vi "rsidr_core_global.vi"() -> ()   [LabVIEW 2020, in "Rohde&Schwarz CMWXP NR FR1 Measurement.lvlib"] (continued)
command(s):\nCONFigure:NRSub:MEAS<i>:MEValuation:LIMit:PDYNamics:OFFPower"}, {"Level"=4, "Class Only"=FALSE, "Identifier"="RSCMWXPNRFR1M_ATTR_MULTI_EVAL_MEAS_LIMIT_POWER_DYNAMICS_TEST_TOLERANCES", "Descriptive Name"="Multi Eval Meas Limit Power Dynamics Test Tolerances", "Data Type"=enum."RawString", "Command"="CONF:NRS:MEAS{instance}:MEV:LIM:PDYN:TTOL:CBGT", "Access"=enum."Read/Write", "Range Table"="", "Read Callback"="", "Write Callback"="", "Range Callback"="", "Check Callback"="", "Rngtable Callback"="", "Coerce Callback"="", "Supported Models"="", "Instrument Options"="", "Check Status Callback"="", "Flags"=0, "Help"="Defines test tolerances for power dynamics limits, for channel BW > 40 MHz.\n\nSyntax:\nCONFigure:NRSub:MEAS<i>:MEValuation:LIMit:PDYNamics:TTOLerance:CBGT <TTPowerLess3G>, <TTPowerGreat3G>\n\n<TTPowerLess3G>\nFor carrier center frequencies up to 3 GHz\nValid Values:\n-3 dB to 3 dB\n\n<TTPowerGreat3G>\nFor carrier center frequencies > 3 GHz\nValid Values:\n-3 dB to 3 dB\n\nAvailable Repeated Capabilities:\ninstance: i0, i1, i2, i3, i4, i5, i6, i7, i8, i9, i10, i11, i12, i13, i14, i15, i16, i17, i18, i19, i20, i21, i22, i23, i24, i25, i26, i27, i28, i29, i30, i31, i32\r\n\nRemote-control command(s):\nCONFigure:NRSub:MEAS<i>:MEValuation:LIMit:PDYNamics:TTOLerance:CBGT"}, {"Level"=4, "Class Only"=FALSE, "Identifier"="RSCMWXPNRFR1M_ATTR_MULTI_EVAL_MEAS_LIMIT_POWER_DYNAMICS_TEST_TOLERANCES_FOR_CHANNEL_BW", "Descriptive Name"="Multi Eval Meas Limit Power Dynamics Test Tolerances For Channel BW", "Data Type"=enum."RawString", "Command"="CONF:NRS:MEAS{instance}:MEV:LIM:PDYN:TTOL:CBLT", "Access"=enum."Read/Write", "Range Table"="", "Read Callback"="", "Write Callback"="", "Range Callback"="", "Check Callback"="", "Rngtable Callback"="", "Coerce Callback"="", "Supported Models"="", "Instrument Options"="", "Check Status Callback"="", "Flags"=0, "Help"="Defines test tolerances for power dynamics limits, for channel BW up to 40 MHz.\n\nSyntax:\nCONFigure:NRSub:MEAS<i>:MEValuation:LIMit:PDYNamics:TTOLerance:CBLT <TTPowerLess3G>, <TTPowerGreat3G>\n\n<TTPowerLess3G>\nFor carrier center frequencies up to 3 GHz\nValid Values:\n-3 dB to 3 dB\n\n<TTPowerGreat3G>\nFor carrier center frequencies > 3 GHz\nValid Values:\n-3 dB to 3 dB\n\nAvailable Repeated Capabilities:\ninstance: i0, i1, i2, i3, i4, i5, i6, i7, i8, i9, i10, i11, i12, i13, i14, i15, i16, i17, i18, i19, i20, i21, i22, i23, i24, i25, i26, i27, i28, i29, i30, i31, i32\r\n\nRemote-control command(s):\nCONFigure:NRSub:MEAS<i>:MEValuation:LIMit:PDYNamics:TTOLerance:CBLT"}, {"Level"=2, "Class Only"=TRUE, "Identifier"="", "Descriptive Name"="Results", "Data Type"=enum."ViInt32", "Command"="", "Access"=enum."Read Only", "Range Table"="", "Read Callback"="", "Write Callback"="", "Range Callback"="", "Check Callback"="", "Rngtable Callback"="", "Coerce Callback"="", "Supported Models"="", "Instrument Options"="", "Check Status Callback"="", "Flags"=0, "Help"="The attributes in this class retrieve results for multi-evaluation measurements."}, {"Level"=3, "Class Only"=TRUE, "Identifier"="", "Descriptive Name"="Detected Signal Configuration", "Data Type"=enum."ViInt32", "Command"="", "Access"=enum."Read Only", "Range Table"="", "Read Callback"="", "Write Callback"="", "Range Callback"="", "Check Callback"="", "Rngtable Callback"="", "Coerce Callback"="", "Supported Models"="", "Instrument Options"="", "Check Status Callback"="", "Flags"=0, "Help"="The commands in this class return the detected allocation and modulation scheme and the view filter throughput."}, {"Level"=4, "Class Only"=FALSE, "Identifier"="RSCMWXPNRFR1M_ATTR_FETCH_MULTI_EVAL_MEAS_MODULATION_DETECTED_ALLOCATION_RESULTS", "Descriptive Name"="Fetch Multi Eval Meas Modulation Detected Allocation Results", "Data Type"=enum."RawString", "Command"="FETC:NRS:MEAS{instance}:MEV:MOD:DALL?", "Access"=enum."Read Only", "Range Table"="", "Read Callback"="", "Write Callback"="", "Range Callback"="", "Check Callback"="", "Rngtable Callback"="", "Coerce Callback"="", "Supported Models"="", "Instrument Options"="", "Check Status Callback"="", "Flags"=0, "Help"="Returns the modulation detected allocation for the measured slot.\n\nIf the same slot is measured by the individual measurements, all commands yield the same result. If different statistic counts are defined for the modulation, ACLR and spectrum emission mask measurements, different slots can be measured and different results can be returned by the individual commands.\n\nReturn values:\n<Reliability>\n decimal\n\n<NrResBlocks>\n decimal\nNumber of allocated resource blocks\n\n<OffsetResBlocks>\n decimal\nOffset of the first allocated resource block from the edge of the allocated UL transmission bandwidth\n\nAvailable Repeated Capabilities:\ninstance: i0, i1, i2, i3, i4, i5, i6, i7, i8, i9, i10, i11, i12, i13, i14, i15, i16, i17, i18, i19, i20, i21, i22, i23, i24, i25, i26, i27, i28, i29, i30, i31, i32\r\n\nRemote-control command(s):\nFETCh:NRSub:MEAS<i>:MEValuation:MODulation:DALLocation?"}, {"Level"=4, "Class Only"=FALSE, "Identifier"="RSCMWXPNRFR1M_ATTR_FETCH_MULTI_EVAL_MEAS_MODULATION_DETECTED_MODULATION_RESULTS", "Descriptive Name"="Fetch Multi Eval Meas Modulation Detected Modulation Results", "Data Type"=enum."RawString", "Command"="FETC:NRS:MEAS{instance}:MEV:MOD:DMOD?", "Access"=enum."Read Only", "Range Table"="", "Read Callback"="", "Write Callback"="", "Range Callback"="", "Check Callback"="", "Rngtable Callback"="", "Coerce Callback"="", "Supported Models"="", "Instrument Options"="", "Check Status Callback"="", "Flags"=0, "Help"="Returns the detected modulation scheme in the measured slot.\n\nReturn values:\n<Reliability>\n decimal\n\n<Modulation>\n BPSK | BPWS | QPSK | Q16 | Q64 | Q256\nBPSK, BPWS: Pi/2-BPSK, Pi/2-BPSK with shaping\nQPSK, Q16, Q64, Q256: QPSK, 16-QAM, 64-QAM, 256-QAM\n\nAvailable Repeated Capabilities:\ninstance: i0, i1, i2, i3, i4, i5, i6, i7, i8, i9, i10, i11, i12, i13, i14, i15, i16, i17, i18, i19, i20, i21, i22, i23, i24, i25, i26, i27, i28, i29, i30, i31, i32\r\n\nRemote-control command(s):\nFETCh:NRSub:MEAS<i>:MEValuation:MODulation:DMODulation?"}, {"Level"=4, "Class Only"=FALSE, "Identifier"="RSCMWXPNRFR1M_ATTR_FETCH_MULTI_EVAL_MEAS_ACLR_DETECTED_ALLOCATION_RESULTS", "Descriptive Name"="Fetch Multi Eval Meas ACLR Detected Allocation Results", "Data Type"=enum."RawString", "Command"="FETC:NRS:MEAS{instance}:MEV:ACLR:DALL?", "Access"=enum."Read Only", "Range Table"="", "Read Callback"="", "Write Callback"="", "Range Callback"="", "Check Callback"="", "Rngtable Callback"="", "Coerce Callback"="", "Supported Models"="", "Instrument Options"="", "Check Status Callback"="", "Flags"=0, "Help"="Returns the ACLR detected allocation for the measured slot.\n\nIf the same slot is measured by the individual measurements, all commands yield the same result. If different statistic counts are defined for the modulation, ACLR and spectrum emission mask measurements, different slots can be measured and different results can be returned by the individual commands.\n\nReturn values:\n<Reliability>\n decimal\n\n<NrResBlocks>\n decimal\nNumber of allocated resource blocks\n\n<OffsetResBlocks>\n decimal\nOffset of the first allocated resource block from the edge of the allocated UL transmission bandwidth\n\nAvailable Repeated Capabilities:\ninstance: i0, i1, i2, i3, i4, i5, i6, i7, i8, i9, i10, i11, i12, i13, i14, i15, i16, i17, i18, i19, i20, i21, i22, i23, i24, i25, i26, i27, i28, i29, i30, i31, i32\r\n\nRemote-control command(s):\nFETCh:NRSub:MEAS<i>:MEValuation:ACLR:DALLocation?"}, {"Level"=4, "Class Only"=FALSE, "Identifier"="RSCMWXPNRFR1M_ATTR_FETCH_MULTI_EVAL_MEAS_SEM_DETECTED_ALLOCATION_RESULTS", "Descriptive Name"="Fetch Multi Eval Meas SEM Detected Allocation Results", "Data Type"=enum."RawString", "Command"="FETC:NRS:MEAS{instance}:MEV:SEM:DALL?", "Access"=enum."Read Only", "Range Table"="", "Read Callback"="", "Write Callback"="", "Range Callback"="", "Check Callback"="", "Rngtable Callback"="", "Coerce Callback"="", "Supported Models"="", "Instrument Options"="", "Check Status Callback"="", "Flags"=0, "Help"="Returns the spectrum emission mask detected allocation for the measured slot.\n\nIf the same slot is measured by the individual measurements, all commands yield the same result. If different statistic counts are defined for the modulation, ACLR and spectrum emission mask measurements, different slots can be measured and different results can be returned by the individual commands.\n\nReturn values:\n<Reliability>\n decimal\n\n<NrResBlocks>\n decimal\nNumber of allocated resource blocks\n\n<OffsetResBlocks>\n decimal\nOffset of the first allocated resource block from the edge of the allocated UL transmission bandwidth\n\nAvailable Repeated Capabilities:\ninstance: i0, i1, i2, i3, i4, i5, i6, i7, i8, i9, i10, i11, i12, i13, i14, i15, i16, i17, i18, i19, i20, i21, i22, i23, i24, i25, i26, i27, i28, i29, i30, i31, i32\r\n\nRemote-control command(s):\nFETCh:NRSub:MEAS<i>:MEValuation:SEMask:DALLocation?"}, {"Level"=4, "Class Only"=FALSE, "Identifier"="RSCMWXPNRFR1M_ATTR_FETCH_MULTI_EVAL_MEAS_VIEW_FILTER_THROUGHPUT", "Descriptive Name"="Fetch Multi Eval Meas View Filter Throughput", "Data Type"=enum."RawString", "Command"="FETC:NRS:MEAS{instance}:MEV:VFTH?", "Access"=enum."Read Only", "Range Table"="", "Read Callback"="", "Write Callback"="", "Range Callback"="", "Check Callback"="", "Rngtable Callback"="", "Coerce Callback"="", "Supported Models"="", "Instrument Options"="", "Check Status Callback"="", "Flags"=0, "Help"="Queries the percentage of measurement intervals in which the detected signal configuration matched the 'View Filter' settings. Only slots which contribute to the 'View Filter Throughput' are displayed, counted, and used for the statistical results. Other slots are rejected.\n\nThe 'View Filter Throughput' is evaluated in a moving window of 1000 frames. If a non-matching signal configuration is changed according to the 'View Filter' settings, the throughput increases linearly from 0% to 100%.\n\n<Reliability>\n decimal\n'Reliability Indicator'\n\n<VFThroughput>\n float\nDefault unit:  %\n\nAvailable Repeated Capabilities:\ninstance: i0, i1, i2, i3, i4, i5, i6, i7, i8, i9, i10, i11, i12, i13, i14, i15, i16, i17, i18, i19, i20, i21, i22, i23, i24, i25, i26, i27, i28, i29, i30, i31, i32\r\n\nRemote-control command(s):\nFETCh:NRSub:MEAS<i>:MEValuation:VFTHroughput?"}, {"Level"=3, "Class Only"=TRUE, "Identifier"="", "Descriptive Name"="EVM Trace Results", "Data Type"=enum."ViInt32", "Command"="", "Access"=enum."Read Only", "Range Table"="", "Read Callback"="", "Write Callback"="", "Range Callback"="", "Check Callback"="", "Rngtable Callback"="", "Coerce Callback"="", "Supported Models"="", "Instrument Options"="", "Check Status Callback"="", "Flags"=0, "Help"="The commands in this class return the contents of the EVM result diagrams."}, {"Level"=4, "Class Only"=FALSE, "Identifier"="RSCMWXPNRFR1M_ATTR_READ_MULTI_EVAL_MEAS_EVM_CURRENT_RESULTS", "Descriptive Name"="Read Multi Eval Meas EVM Current Results", "Data Type"=enum."RawString", "Command"="READ:NRS:MEAS{instance}:MEV:EVM:CURR?", "Access"=enum."Read Only", "Range Table"="", "Read Callback"="", "Write Callback"="", "Range Callback"="", "Check Callback"="", "Rngtable Callback"="", "Coerce Callback"="", "Supported Models"="", "Instrument Options"="", "Check Status Callback"="", "Flags"=0, "Help"="Returns the values of the EVM RMS bar graphs for the OFDM symbols in the measured slot. The results of the current bar graph are retrieved.\n\nThere is one pair of EVM values per OFDM symbol, returned in the following order:\n<Reliability>, {<Low>, <High>}symbol 0, {<Low>, <High>}symbol 1, ...\n\nReturn values:\n<Reliability>\n decimal\n\n<Low>\n float\nEVM value for low EVM window position.\nDefault unit:  %\n\n<High>\n float\nEVM value for high EVM window position.\nDefault unit:  %\n\nAvailable Repeated Capabilities:\ninstance: i0, i1, i2, i3, i4, i5, i6, i7, i8, i9, i10, i11, i12, i13, i14, i15, i16, i17, i18, i19, i20, i21, i22, i23, i24, i25, i26, i27, i28, i29, i30, i31, i32\r\n\nRemote-control command(s):\nREAD:NRSub:MEAS<i>:MEValuation:EVMagnitude:CURRent?"}, {"Level"=4, "Class Only"=FALSE, "Identifier"="RSCMWXPNRFR1M_ATTR_READ_MULTI_EVAL_MEAS_EVM_AVERAGE_RESULTS", "Descriptive Name"="Read Multi Eval Meas EVM Average Results", "Data Type"=enum."RawString", "Command"="READ:NRS:MEAS{instance}:MEV:EVM:AVER?", "Access"=enum."Read Only", "Range Table"="", "Read Callback"="", "Write Callback"="", "Range Callback"="", "Check Callback"="", "Rngtable Callback"="", "Coerce Callback"="", "Supported Models"="", "Instrument Options"="", "Check Status Callback"="", "Flags"=0, "Help"="Returns the values of the EVM RMS bar graphs for the OFDM symbols in the measured slot. The results of the average  bar graph are retrieved.\n\nThere is one pair of EVM values per OFDM symbol, returned in the following order:\n<Reliability>, {<Low>, <High>}symbol 0, {<Low>, <High>}symbol 1, ...\n\nReturn values:\n<Reliability>\n decimal\n\n<Low>\n float\nEVM value for low EVM window position.\nDefault unit:  %\n\n<High>\n float\nEVM value for high EVM window position.\nDefault unit:  %\n\nAvailable Repeated Capabilities:\ninstance: i0, i1, i2, i3, i4, i5, i6, i7, i8, i9, i10, i11, i12, i13, i14, i15, i16, i17, i18, i19, i20, i21, i22, i23, i24, i25, i26, i27, i28, i29, i30, i31, i32\r\n\nRemote-control command(s):\nREAD:NRSub:MEAS<i>:MEValuation:EVMagnitude:AVERage?"}, {"Level"=4, "Class Only"=FALSE, "Identifier"="RSCMWXPNRFR1M_ATTR_READ_MULTI_EVAL_MEAS_EVM_MAXIMUM_RESULTS", "Descriptive Name"="Read Multi Eval Meas EVM Maximum Results", "Data Type"=enum."RawString", "Command"="READ:NRS:MEAS{instance}:MEV:EVM:MAX?", "Access"=enum."Read Only", "Range Table"="", "Read Callback"="", "Write Callback"="", "Range Callback"="", "Check Callback"="", "Rngtable Callback"="", "Coerce Callback"="", "Supported Models"="", "Instrument Options"="", "Check Status Callback"="", "Flags"=0, "Help"="Returns the values of the EVM RMS bar graphs for the OFDM symbols in the measured slot. The results of the maximum bar graph are retrieved.\n\nThere is one pair of EVM values per OFDM symbol, returned in the following order:\n<Reliability>, {<Low>, <High>}symbol 0, {<Low>, <High>}symbol 1, ...\n\nReturn values:\n<Reliability>\n decimal\n\n<Low>\n float\nEVM value for low EVM window position.\nDefault unit:  %\n\n<High>\n float\nEVM value for high EVM window position.\nDefault unit:  %\n\nAvailable Repeated Capabilities:\ninstance: i0, i1, i2, i3, i4, i5, i6, i7, i8, i9, i10, i11, i12, i13, i14, i15, i16, i17, i18, i19, i20, i21, i22, i23, i24, i25, i26, i27, i28, i29, i30, i31, i32\r\n\nRemote-control command(s):\nREAD:NRSub:MEAS<i>:MEValuation:EVMagnitude:MAXimum?"}, {"Level"=4, "Class Only"=FALSE, "Identifier"="RSCMWXPNRFR1M_ATTR_FETCH_MULTI_EVAL_MEAS_EVM_CURRENT_RESULTS", "Descriptive Name"="Fetch Multi Eval Meas EVM Current Results", "Data Type"=enum."RawString", "Command"="FETC:NRS:MEAS{instance}:MEV:EVM:CURR?", "Access"=enum."Read Only", "Range Table"="", "Read Callback"="", "Write Callback"="", "Range Callback"="", "Check Callback"="", "Rngtable Callback"="", "Coerce Callback"="", "Supported Models"="", "Instrument Options"="", "Check Status Callback"="", "Flags"=0, "Help"="Returns the values of the EVM RMS bar graphs for the OFDM symbols in the measured slot. The results of the current bar graph are retrieved.\n\nThere is one pair of EVM values per OFDM symbol, returned in the following order:\n<Reliability>, {<Low>, <High>}symbol 0, {<Low>, <High>}symbol 1, ...\n\nReturn values:\n<Reliability>\n decimal\n\n<Low>\n float\nEVM value for low EVM window position.\nDefault unit:  %\n\n<High>\n float\nEVM value for high EVM window position.\nDefault unit:  %\n\nAvailable Repeated Capabilities:\ninstance: i0, i1, i2, i3, i4, i5, i6, i7, i8, i9, i10, i11, i12, i13, i14, i15, i16, i17, i18, i19, i20, i21, i22, i23, i24, i25, i26, i27, i28, i29, i30, i31, i32\r\n\nRemote-control command(s):\nFETCh:NRSub:MEAS<i>:MEValuation:EVMagnitude:CURRent?"}, {"Level"=4, "Class Only"=FALSE, "Identifier"="RSCMWXPNRFR1M_ATTR_FETCH_MULTI_EVAL_MEAS_EVM_AVERAGE_RESULTS", "Descriptive Name"="Fetch Multi Eval Meas EVM Average Results", "Data Type"=enum."RawString", "Command"="FETC:NRS:MEAS{instance}:MEV:EVM:AVER?", "Access"=enum."Read Only", "Range Table"="", "Read Callback"="", "Write Callback"="", "Range Callback"="", "Check Callback"="", "Rngtable Callback"="", "Coerce Callback"="", "Supported Models"="", "Instrument Options"="", "Check Status Callback"="", "Flags"=0, "Help"="Returns the values of the EVM RMS bar graphs for the OFDM symbols in the measured slot. The results of the average  bar graph are retrieved.\n\nThere is one pair of EVM values per OFDM symbol, returned in the following order:\n<Reliability>, {<Low>, <High>}symbol 0, {<Low>, <High>}symbol 1, ...\n\nReturn values:\n<Reliability>\n decimal\n\n<Low>\n float\nEVM value for low EVM window position.\nDefault unit:  %\n\n<High>\n float\nEVM value for high EVM window position.\nDefault unit:  %\n\nAvailable Repeated Capabilities:\ninstance: i0, i1, i2, i3, i4, i5, i6, i7, i8, i9, i10, i11, i12, i13, i14, i15, i16, i17, i18, i19, i20, i21, i22, i23, i24, i25, i26, i27, i28, i29, i30, i31, i32\r\n\nRemote-control command(s):\nFETCh:NRSub:MEAS<i>:MEValuation:EVMagnitude:AVERage?"}, {"Level"=4, "Class Only"=FALSE, "Identifier"="RSCMWXPNRFR1M_ATTR_FETCH_MULTI_EVAL_MEAS_EVM_MAXIMUM_RESULTS", "Descriptive Name"="Fetch Multi Eval Meas EVM Maximum Results", "Data Type"=enum."RawString", "Command"="FETC:NRS:MEAS{instance}:MEV:EVM:MAX?", "Access"=enum."Read Only", "Range Table"="", "Read Callback"="", "Write Callback"="", "Range Callback"="", "Check Callback"="", "Rngtable Callback"="", "Coerce Callback"="", "Supported Models"="", "Instrument Options"="", "Check Status Callback"="", "Flags"=0, "Help"="Returns the values of the EVM RMS bar graphs for the OFDM symbols in the measured slot. The results of the maximum bar graph are retrieved.\n\nThere is one pair of EVM values per OFDM symbol, returned in the following order:\n<Reliability>, {<Low>, <High>}symbol 0, {<Low>, <High>}symbol 1, ...\n\nReturn values:\n<Reliability>\n decimal\n\n<Low>\n float\nEVM value for low EVM window position.\nDefault unit:  %\n\n<High>\n float\nEVM value for high EVM window position.\nDefault unit:  %\n\nAvailable Repeated Capabilities:\ninstance: i0, i1, i2, i3, i4, i5, i6, i7, i8, i9, i10, i11, i12, i13, i14, i15, i16, i17, i18, i19, i20, i21, i22, i23, i24, i25, i26, i27, i28, i29, i30, i31, i32\r\n\nRemote-control command(s):\nFETCh:NRSub:MEAS<i>:MEValuation:EVMagnitude:MAXimum?"}, {"Level"=4, "Class Only"=FALSE, "Identifier"="RSCMWXPNRFR1M_ATTR_READ_MULTI_EVAL_MEAS_EVM_PEAK_CURRENT_RESULTS", "Descriptive Name"="Read Multi Eval Meas EVM Peak Current Results", "Data Type"=enum."RawString", "Command"="READ:NRS:MEAS{instance}:MEV:EVM:PEAK:CURR?", "Access"=enum."Read Only", "Range Table"="", "Read Callback"="", "Write Callback"="", "Range Callback"="", "Check Callback"="", "Rngtable Callback"="", "Coerce Callback"="", "Supported Models"="", "Instrument Options"="", "Check Status Callback"="", "Flags"=0, "Help"="Returns the values of the EVM peak bar graphs for the OFDM symbols in the measured slot. The results of the current bar graph are retrieved.\n\nThere is one pair of EVM values per OFDM symbol, returned in the following order:\n<Reliability>, {<Low>, <High>}symbol 0, {<Low>, <High>}symbol 1, ...\n\nReturn values:\n<Reliability>\n decimal\n\n<Low>\n float\nEVM value for low EVM window position.\nDefault unit:  %\n\n<High>\n float\nEVM value for high EVM window position.\nDefault unit:  %\n\nAvailable Repeated Capabilities:\ninstance: i0, i1, i2, i3, i4, i5, i6, i7, i8, i9, i10, i11, i12, i13, i14, i15, i16, i17, i18, i19, i20, i21, i22, i23, i24, i25, i26, i27, i28, i29, i30, i31, i32\r\n\nRemote-control command(s):\nREAD:NRSub:MEAS<i>:MEValuation:EVMagnitude:PEAK:CURRent?"}, {"Level"=4, "Class Only"=FALSE, "Identifier"="RSCMWXPNRFR1M_ATTR_READ_MULTI_EVAL_MEAS_EVM_PEAK_AVERAGE_RESULTS", "Descriptive Name"="Read Multi Eval Meas EVM Peak Average Results", "Data Type"=enum."RawString", "Command"="READ:NRS:MEAS{instance}:MEV:EVM:PEAK:AVER?", "Access"=enum."Read Only", "Range Table"="", "Read Callback"="", "Write Callback"="", "Range Callback"="", "Check Callback"="", "Rngtable Callback"="", "Coerce Callback"="", "Supported Models"="", "Instrument Options"="", "Check Status Callback"="", "Flags"=0, "Help"="Returns the values of the EVM peak bar graphs for the OFDM symbols in the measured slot. The results of the average bar graph are retrieved.\n\nThere is one pair of EVM values per OFDM symbol, returned in the following order:\n<Reliability>, {<Low>, <High>}symbol 0, {<Low>, <High>}symbol 1, ...\n\nReturn values:\n<Reliability>\n decimal\n\n<Low>\n float\nEVM value for low EVM window position.\nDefault unit:  %\n\n<High>\n float\nEVM value for high EVM window position.\nDefault unit:  %\n\nAvailable Repeated Capabilities:\ninstance: i0, i1, i2, i3, i4, i5, i6, i7, i8, i9, i10, i11, i12, i13, i14, i15, i16, i17, i18, i19, i20, i21, i22, i23, i24, i25, i26, i27, i28, i29, i30, i31, i32\r\n\nRemote-control command(s):\nREAD:NRSub:MEAS<i>:MEValuation:EVMagnitude:PEAK:AVERage?"}, {"Level"=4, "Class Only"=FALSE, "Identifier"="RSCMWXPNRFR1M_ATTR_READ_MULTI_EVAL_MEAS_EVM_PEAK_MAXIMUM_RESULTS", "Descriptive Name"="Read Multi Eval Meas EVM Peak Maximum Results", "Data Type"=enum."RawString", "Command"="READ:NRS:MEAS{instance}:MEV:EVM:PEAK:MAX?", "Access"=enum."Read Only", "Range Table"="", "Read Callback"="", "Write Callback"="", "Range Callback"="", "Check Callback"="", "Rngtable Callback"="", "Coerce Callback"="", "Supported Models"="", "Instrument Options"="", "Check Status Callback"="", "Flags"=0, "Help"="Returns the values of the EVM peak bar graphs for the OFDM symbols in the measured slot. The results of the maximum bar graph are retrieved.\n\nThere is one pair of EVM values per OFDM symbol, returned in the following order:\n<Reliability>, {<Low>, <High>}symbol 0, {<Low>, <High>}symbol 1, ...\n\nReturn values:\n<Reliability>\n decimal\n\n<Low>\n float\nEVM value for low EVM window position.\nDefault unit:  %\n\n<High>\n float\nEVM value for high EVM window position.\nDefault unit:  %\n\nAvailable Repeated Capabilities:\ninstance: i0, i1, i2, i3, i4, i5, i6, i7, i8, i9, i10, i11, i12, i13, i14, i15, i16, i17, i18, i19, i20, i21, i22, i23, i24, i25, i26, i27, i28, i29, i30, i31, i32\r\n\nRemote-control command(s):\nREAD:NRSub:MEAS<i>:MEValuation:EVMagnitude:PEAK:MAXimum?"}, {"Level"=4, "Class Only"=FALSE, "Identifier"="RSCMWXPNRFR1M_ATTR_FETCH_MULTI_EVAL_MEAS_EVM_PEAK_CURRENT_RESULTS", "Descriptive Name"="Fetch Multi Eval Meas EVM Peak Current Results", "Data Type"=enum."RawString", "Command"="FETC:NRS:MEAS{instance}:MEV:EVM:PEAK:CURR?", "Access"=enum."Read Only", "Range Table"="", "Read Callback"="", "Write Callback"="", "Range Callback"="", "Check Callback"="", "Rngtable Callback"="", "Coerce Callback"="", "Supported Models"="", "Instrument Options"="", "Check Status Callback"="", "Flags"=0, "Help"="Returns the values of the EVM peak bar graphs for the OFDM symbols in the measured slot. The results of the current bar graph are retrieved.\n\nThere is one pair of EVM values per OFDM symbol, returned in the following order:\n<Reliability>, {<Low>, <High>}symbol 0, {<Low>, <High>}symbol 1, ...\n\nReturn values:\n<Reliability>\n decimal\n\n<Low>\n float\nEVM value for low EVM window position.\nDefault unit:  %\n\n<High>\n float\nEVM value for high EVM window position.\nDefault unit:  %\n\nAvailable Repeated Capabilities:\ninstance: i0, i1, i2, i3, i4, i5, i6, i7, i8, i9, i10, i11, i12, i13, i14, i15, i16, i17, i18, i19, i20, i21, i22, i23, i24, i25, i26, i27, i28, i29, i30, i31, i32\r\n\nRemote-control command(s):\nFETCh:NRSub:MEAS<i>:MEValuation:EVMagnitude:PEAK:CURRent?"}, {"Level"=4, "Class Only"=FALSE, "Identifier"="RSCMWXPNRFR1M_ATTR_FETCH_MULTI_EVAL_MEAS_EVM_PEAK_AVERAGE_RESULTS", "Descriptive Name"="Fetch Multi Eval Meas EVM Peak Average Results", "Data Type"=enum."RawString", "Command"="FETC:NRS:MEAS{instance}:MEV:EVM:PEAK:AVER?", "Access"=enum."Read Only", "Range Table"="", "Read Callback"="", "Write Callback"="", "Range Callback"="", "Check Callback"="", "Rngtable Callback"="", "Coerce Callback"="", "Supported Models"="", "Instrument Options"="", "Check Status Callback"="", "Flags"=0, "Help"="Returns the values of the EVM peak bar graphs for the OFDM symbols in the measured slot. The results of the average bar graph are retrieved.\n\nThere is one pair of EVM values per OFDM symbol, returned in the following order:\n<Reliability>, {<Low>, <High>}symbol 0, {<Low>, <High>}symbol 1, ...\n\nReturn values:\n<Reliability>\n decimal\n\n<Low>\n float\nEVM value for low EVM window position.\nDefault unit:  %\n\n<High>\n float\nEVM value for high EVM window position.\nDefault unit:  %\n\nAvailable Repeated Capabilities:\ninstance: i0, i1, i2, i3, i4, i5, i6, i7, i8, i9, i10, i11, i12, i13, i14, i15, i16, i17, i18, i19, i20, i21, i22, i23, i24, i25, i26, i27, i28, i29, i30, i31, i32\r\n\nRemote-control command(s):\nFETCh:NRSub:MEAS<i>:MEValuation:EVMagnitude:PEAK:AVERage?"}, {"Level"=4, "Class Only"=FALSE, "Identifier"="RSCMWXPNRFR1M_ATTR_FETCH_MULTI_EVAL_MEAS_EVM_PEAK_MAXIMUM_RESULTS", "Descriptive Name"="Fetch Multi Eval Meas EVM Peak Maximum Results", "Data Type"=enum."RawString", "Command"="FETC:NRS:MEAS{instance}:MEV:EVM:PEAK:MAX?", "Access"=enum."Read Only", "Range Table"="", "Read Callback"="", "Write Callback"="", "Range Callback"="", "Check Callback"="", "Rngtable Callback"="", "Coerce Callback"="", "Supported Models"="", "Instrument Options"="", "Check Status Callback"="", "Flags"=0, "Help"="Returns the values of the EVM peak bar graphs for the OFDM symbols in the measured slot. The results of the maximum bar graph are retrieved.\n\nThere is one pair of EVM values per OFDM symbol, returned in the following order:\n<Reliability>, {<Low>, <High>}symbol 0, {<Low>, <High>}symbol 1, ...\n\nReturn values:\n<Reliability>\n decimal\n\n<Low>\n float\nEVM value for low EVM window position.\nDefault unit:  %\n\n<High>\n float\nEVM value for high EVM window position.\nDefault unit:  %\n\nAvailable Repeated Capabilities:\ninstance: i0, i1, i2, i3, i4, i5, i6, i7, i8, i9, i10, i11, i12, i13, i14, i15, i16, i17, i18, i19, i20, i21, i22, i23, i24, i25, i26, i27, i28, i29, i30, i31, i32\r\n\nRemote-control command(s):\nFETCh:NRSub:MEAS<i>:MEValuation:EVMagnitude:PEAK:MAXimum?"}, {"Level"=4, "Class Only"=FALSE, "Identifier"="RSCMWXPNRFR1M_ATTR_READ_MULTI_EVAL_MEAS_EVM_VS_SYMBOL_CURRENT_RESULTS", "Descriptive Name"="Read Multi Eval Meas Trace EVM vs Symbol Current Results", "Data Type"=enum."RawString", "Command"="READ:NRS:MEAS{instance}:MEV:TRAC:EVMS:CURR?", "Access"=enum."Read Only", "Range Table"="", "Read Callback"="", "Write Callback"="", "Range Callback"="", "Check Callback"="", "Rngtable Callback"="", "Coerce Callback"="", "Supported Models"="", "Instrument Options"="", "Check Status Callback"="", "Flags"=0, "Help"="Returns the current values of the EVM vs modulation symbol trace.\n\nReturn values:\n<Reliability>\n decimal\n\n<Ratio>\n float\nComma-separated list of EVM values, one value per modulation symbol\nDefault unit:  %\n\nAvailable Repeated Capabilities:\ninstance: i0, i1, i2, i3, i4, i5, i6, i7, i8, i9, i10, i11, i12, i13, i14, i15, i16, i17, i18, i19, i20, i21, i22, i23, i24, i25, i26, i27, i28, i29, i30, i31, i32\r\n\nRemote-control command(s):\nREAD:NRSub:MEAS<i>:MEValuation:TRACe:EVMSymbol:CURRent?"}, {"Level"=4, "Class Only"=FALSE, "Identifier"="RSCMWXPNRFR1M_ATTR_READ_MULTI_EVAL_MEAS_EVM_VS_SYMBOL_AVERAGE_RESULTS", "Descriptive Name"="Read Multi Eval Meas Trace EVM vs Symbol Average Results", "Data Type"=enum."RawString", "Command"="READ:NRS:MEAS{instance}:MEV:TRAC:EVMS:AVER?", "Access"=enum."Read Only", "Range Table"="", "Read Callback"="", "Write Callback"="", "Range Callback"="", "Check Callback"="", "Rngtable Callback"="", "Coerce Callback"="", "Supported Models"="", "Instrument Options"="", "Check Status Callback"="", "Flags"=0, "Help"="Returns the average values of the EVM vs modulation symbol trace.\n\nReturn values:\n<Reliability>\n decimal\n\n<Ratio>\n float\nComma-separated list of EVM values, one value per modulation symbol\nDefault unit:  %\n\nAvailable Repeated Capabilities:\ninstance: i0, i1, i2, i3, i4, i5, i6, i7, i8, i9, i10, i11, i12, i13, i14, i15, i16, i17, i18, i19, i20, i21, i22, i23, i24, i25, i26, i27, i28, i29, i30, i31, i32\r\n\nRemote-control command(s):\nREAD:NRSub:MEAS<i>:MEValuation:TRACe:EVMSymbol:AVERage?"}, {"Level"=4, "Class Only"=FALSE, "Identifier"="RSCMWXPNRFR1M_ATTR_READ_MULTI_EVAL_MEAS_EVM_VS_SYMBOL_MAXIMUM_RESULTS", "Descriptive Name"="Read Multi Eval Meas Trace EVM vs Symbol Maximum Results", "Data Type"=enum."RawString", "Command"="READ:NRS:MEAS{instance}:MEV:TRAC:EVMS:MAX?", "Access"=enum."Read Only", "Range Table"="", "Read Callback"="", "Write Callback"="", "Range Callback"="", "Check Callback"="", "Rngtable Callback"="", "Coerce Callback"="", "Supported Models"="", "Instrument Options"="", "Check Status Callback"="", "Flags"=0, "Help"="Returns the maximum values of the EVM vs modulation symbol trace.\n\nReturn values:\n<Reliability>\n decimal\n\n<Ratio>\n float\nComma-separated list of EVM values, one value per modulation symbol\nDefault unit:  %\n\nAvailable Repeated Capabilities:\ninstance: i0, i1, i2, i3, i4, i5, i6, i7, i8, i9, i10, i11, i12, i13, i14, i15, i16, i17, i18, i19, i20, i21, i22, i23, i24, i25, i26, i27, i28, i29, i30, i31, i32\r\n\nRemote-control command(s):\nREAD:NRSub:MEAS<i>:MEValuation:TRACe:EVMSymbol:MAXimum?"}, {"Level"=4, "Class Only"=FALSE, "Identifier"="RSCMWXPNRFR1M_ATTR_FETCH_MULTI_EVAL_MEAS_EVM_VS_SYMBOL_CURRENT_RESULTS", "Descriptive Name"="Fetch Multi Eval Meas Trace EVM vs Symbol Current Results", "Data Type"=enum."RawString", "Command"="FETC:NRS:MEAS{instance}:MEV:TRAC:EVMS:CURR?", "Access"=enum."Read Only", "Range Table"="", "Read Callback"="", "Write Callback"="", "Range Callback"="", "Check Callback"="", "Rngtable Callback"="", "Coerce Callback"="", "Supported Models"="", "Instrument Options"="", "Check Status Callback"="", "Flags"=0, "Help"="Returns the current values of the EVM vs modulation symbol trace.\n\nReturn values:\n<Reliability>\n decimal\n\n<Ratio>\n float\nComma-separated list of EVM values, one value per modulation symbol\nDefault unit:  %\n\nAvailable Repeated Capabilities:\ninstance: i0, i1, i2, i3, i4, i5, i6, i7, i8, i9, i10, i11, i12, i13, i14, i15, i16, i17, i18, i19, i20, i21, i22, i23, i24, i25, i26, i27, i28, i29, i30, i31, i32\r\n\nRemote-control command(s):\nFETCh:NRSub:MEAS<i>:MEValuation:TRACe:EVMSymbol:CURRent?"}, {"Level"=4, "Class Only"=FALSE, "Identifier"="RSCMWXPNRFR1M_ATTR_FETCH_MULTI_EVAL_MEAS_EVM_VS_SYMBOL_AVERAGE_RESULTS", "Descriptive Name"="Fetch Multi Eval Meas Trace EVM vs Symbol Average Results", "Data Type"=enum."RawString", "Command"="FETC:NRS:MEAS{instance}:MEV:TRAC:EVMS:AVER?", "Access"=enum."Read Only", "Range Table"="", "Read Callback"="", "Write Callback"="", "Range Callback"="", "Check Callback"="", "Rngtable Callback"="", "Coerce Callback"="", "Supported Models"="", "Instrument Options"="", "Check Status Callback"="", "Flags"=0, "Help"="Returns the average values of the EVM vs modulation symbol trace.\n\nReturn values:\n<Reliability>\n decimal\n\n<Ratio>\n float\nComma-separated list of EVM values, one value per modulation symbol\nDefault unit:  %\n\nAvailable Repeated Capabilities:\ninstance: i0, i1, i2, i3, i4, i5, i6, i7, i8, i9, i10, i11, i12, i13, i14, i15, i16, i17, i18, i19, i20, i21, i22, i23, i24, i25, i26, i27, i28, i29, i30, i31, i32\r\n\nRemote-control command(s):\nFETCh:NRSub:MEAS<i>:MEValuation:TRACe:EVMSymbol:AVERage?"}, {"Level"=4, "Class Only"=FALSE, "Identifier"="RSCMWXPNRFR1M_ATTR_FETCH_MULTI_EVAL_MEAS_EVM_VS_SYMBOL_MAXIMUM_RESULTS", "Descriptive Name"="Fetch Multi Eval Meas Trace EVM vs Symbol Maximum Results", "Data Type"=enum."RawString", "Command"="FETC:NRS:MEAS{instance}:MEV:TRAC:EVMS:MAX?", "Access"=enum."Read Only", "Range Table"="", "Read Callback"="", "Write Callback"="", "Range Callback"="", "Check Callback"="", "Rngtable Callback"="", "Coerce Callback"="", "Supported Models"="", "Instrument Options"="", "Check Status Callback"="", "Flags"=0, "Help"="Returns the maximum values of the EVM vs modulation symbol trace.\n\nReturn values:\n<Reliability>\n decimal\n\n<Ratio>\n float\nComma-separated list of EVM values, one value per modulation symbol\nDefault unit:  %\n\nAvailable Repeated Capabilities:\ninstance: i0, i1, i2, i3, i4, i5, i6, i7, i8, i9, i10, i11, i12, i13, i14, i15, i16, i17, i18, i19, i20, i21, i22, i23, i24, i25, i26, i27, i28, i29, i30, i31, i32\r\n\nRemote-control command(s):\nFETCh:NRSub:MEAS<i>:MEValuation:TRACe:EVMSymbol:MAXimum?"}, {"Level"=4, "Class Only"=FALSE, "Identifier"="RSCMWXPNRFR1M_ATTR_READ_MULTI_EVAL_MEAS_TRACE_EVM_VS_SUBCARRIER_RESULTS", "Descriptive Name"="Read Multi Eval Meas Trace EVM vs Subcarrier Results", "Data Type"=enum."RawString", "Command"="READ:NRS:MEAS{instance}:MEV:TRAC:EVMC?", "Access"=enum."Read Only", "Range Table"="", "Read Callback"="", "Write Callback"="", "Range Callback"="", "Check Callback"="", "Rngtable Callback"="", "Coerce Callback"="", "Supported Models"="", "Instrument Options"="", "Check Status Callback"="", "Flags"=0, "Help"="Returns the values of the EVM vs subcarrier trace.\n\nReturn values:\n<Reliability>\n decimal\n\n<Ratio>\n float\nComma-separated list of EVM values, one value per subcarrier\nFor not allocated subcarriers, NCAP is returned.\nDefault unit:  %\n\nAvailable Repeated Capabilities:\ninstance: i0, i1, i2, i3, i4, i5, i6, i7, i8, i9, i10, i11, i12, i13, i14, i15, i16, i17, i18, i19, i20, i21, i22, i23, i24, i25, i26, i27, i28, i29, i30, i31, i32\r\n\nRemote-control command(s):\nREAD:NRSub:MEAS<i>:MEValuation:TRACe:EVMC?"}, {"Level"=4, "Class Only"=FALSE, "Identifier"="RSCMWXPNRFR1M_ATTR_FETCH_MULTI_EVAL_MEAS_TRACE_EVM_VS_SUBCARRIER_RESULTS", "Descriptive Name"="Fetch Multi Eval Meas Trace EVM vs Subcarrier Results", "Data Type"=enum."RawString", "Command"="FETC:NRS:MEAS{instance}:MEV:TRAC:EVMC?", "Access"=enum."Read Only", "Range Table"="", "Read Callback"="", "Write Callback"="", "Range Callback"="", "Check Callback"="", "Rngtable Callback"="", "Coerce Callback"="", "Supported Models"="", "Instrument Options"="", "Check Status Callback"="", "Flags"=0, "Help"="Returns the values of the EVM vs subcarrier trace.\n\nReturn values:\n<Reliability>\n decimal\n\n<Ratio>\n float\nComma-separated list of EVM values, one value per subcarrier\nFor not allocated subcarriers, NCAP is returned.\nDefault unit:  %\n\nAvailable Repeated Capabilities:\ninstance: i0, i1, i2, i3, i4, i5, i6, i7, i8, i9, i10, i11, i12, i13, i14, i15, i16, i17, i18, i19, i20, i21, i22, i23, i24, i25, i26, i27, i28, i29, i30, i31, i32\r\n\nRemote-control command(s):\nFETCh:NRSub:MEAS<i>:MEValuation:TRACe:EVMC?"}, {"Level"=3, "Class Only"=TRUE, "Identifier"="", "Descriptive Name"="Magnitude Error", "Data Type"=enum."ViInt32", "Command"="", "Access"=enum."Read Only", "Range Table"="", "Read Callback"="", "Write Callback"="", "Range Callback"="", "Check Callback"="", "Rngtable Callback"="", "Coerce Callback"="", "Supported Models"="", "Instrument Options"="", "Check Status Callback"="", "Flags"=0, "Help"="The commands in this class return the contents of the magnitude error vs OFDM symbol result diagram."}, {"Level"=4, "Class Only"=FALSE, "Identifier"="RSCMWXPNRFR1M_ATTR_READ_MULTI_EVAL_MEAS_MAGNITUDE_ERROR_CURRENT_RESULTS", "Descriptive Name"="Read Multi Eval Meas Magnitude Error Current Results", "Data Type"=enum."RawString", "Command"="READ:NRS:MEAS{instance}:MEV:MERR:CURR?", "Access"=enum."Read Only", "Range Table"="", "Read Callback"="", "Write Callback"="", "Range Callback"="", "Check Callback"="", "Rngtable Callback"="", "Coerce Callback"="", "Supported Models"="", "Instrument Options"="", "Check Status Callback"="", "Flags"=0, "Help"="Returns the values of the magnitude error bar graphs for the OFDM symbols in the measured slot. The results of the current bar graph are retrieved.\nThere is one pair of magnitude error values per OFDM symbol, returned in the following order:\n<Reliability>, {<Low>, <High>}symbol 0, {<Low>, <High>}symbol 1, ...\n\nReturn values:\n<Reliability>\n decimal\n\n<Low>\n float\nMagnitude error value for low EVM window position.\nDefault unit:  %\n\n<High>\n float\nMagnitude error value for high EVM window position.\nDefault unit:  %\n\nAvailable Repeated Capabilities:\ninstance: i0, i1, i2, i3, i4, i5, i6, i7, i8, i9, i10, i11, i12, i13, i14, i15, i16, i17, i18, i19, i20, i21, i22, i23, i24, i25, i26, i27, i28, i29, i30, i31, i32\r\n\nRemote-control command(s):\nREAD:NRSub:MEAS<i>:MEValuation:MERRor:CURRent?"}, {"Level"=4, "Class Only"=FALSE, "Identifier"="RSCMWXPNRFR1M_ATTR_READ_MULTI_EVAL_MEAS_MAGNITUDE_ERROR_AVERAGE_RESULTS", "Descriptive Name"="Read Multi Eval Meas Magnitude Error Average Results", "Data Type"=enum."RawString", "Command"="READ:NRS:MEAS{instance}:MEV:MERR:AVER?", "Access"=enum."Read Only", "Range Table"="", "Read Callback"="", "Write Callback"="", "Range Callback"="", "Check Callback"="", "Rngtable Callback"="", "Coerce Callback"="", "Supported Models"="", "Instrument Options"="", "Check Status Callback"="", "Flags"=0, "Help"="Returns the values of the magnitude error bar graphs for the OFDM symbols in the measured slot. The results of the average bar graph are retrieved.\nThere is one pair of magnitude error values per OFDM symbol, returned in the following order:\n<Reliability>, {<Low>, <High>}symbol 0, {<Low>, <High>}symbol 1, ...\n\nReturn values:\n<Reliability>\n decimal\n\n<Low>\n float\nMagnitude error value for low EVM window position.\nDefault unit:  %\n\n<High>\n float\nMagnitude error value for high EVM window position.\nDefault unit:  %\n\nAvailable Repeated Capabilities:\ninstance: i0, i1, i2, i3, i4, i5, i6, i7, i8, i9, i10, i11, i12, i13, i14, i15, i16, i17, i18, i19, i20, i21, i22, i23, i24, i25, i26, i27, i28, i29, i30, i31, i32\r\n\nRemote-control command(s):\nREAD:NRSub:MEAS<i>:MEValuation:MERRor:AVERage?"}, {"Level"=4, "Class Only"=FALSE, "Identifier"="RSCMWXPNRFR1M_ATTR_READ_MULTI_EVAL_MEAS_MAGNITUDE_ERROR_MAXIMUM_RESULTS", "Descriptive Name"="Read Multi Eval Meas Magnitude Error Maximum Results", "Data Type"=enum."RawString", "Command"="READ:NRS:MEAS{instance}:MEV:MERR:MAX?", "Access"=enum."Read Only", "Range Table"="", "Read Callback"="", "Write Callback"="", "Range Callback"="", "Check Callback"="", "Rngtable Callback"="", "Coerce Callback"="", "Supported Models"="", "Instrument Options"="", "Check Status Callback"="", "Flags"=0, "Help"="Returns the values of the magnitude error bar graphs for the OFDM symbols in the measured slot. The results of the maximum bar graph are retrieved.\nThere is one pair of magnitude error values per OFDM symbol, returned in the following order:\n<Reliability>, {<Low>, <High>}symbol 0, {<Low>, <High>}symbol 1, ...\n\nReturn values:\n<Reliability>\n decimal\n\n<Low>\n float\nMagnitude error value for low EVM window position.\nDefault unit:  %\n\n<High>\n float\nMagnitude error value for high EVM window position.\nDefault unit:  %\n\nAvailable Repeated Capabilities:\ninstance: i0, i1, i2, i3, i4, i5, i6, i7, i8, i9, i10, i11, i12, i13, i14, i15, i16, i17, i18, i19, i20, i21, i22, i23, i24, i25, i26, i27, i28, i29, i30, i31, i32\r\n\nRemote-control command(s):\nREAD:NRSub:MEAS<i>:MEValuation:MERRor:MAXimum?"}, {"Level"=4, "Class Only"=FALSE, "Identifier"="RSCMWXPNRFR1M_ATTR_FETCH_MULTI_EVAL_MEAS_MAGNITUDE_ERROR_CURRENT_RESULTS", "Descriptive Name"="Fetch Multi Eval Meas Magnitude Error Current Results", "Data Type"=enum."RawString", 
